vi "Set_tdms_properties.vi"(8 "Measurement Duration(s)":dbl=30.0 caption="Measurement Duration" format="%.3g", 11 "Temperature":string) -> (2 "Property Values":string[](array[string]), 3 "property names":string[](array[string])=["Temperature", "HV", "LV", "CH1 V/Div", "CH2 V/Div", "Trigger Level", "Trigger Source", "Coincidence"])   [LabVIEW 2019]
uses:
  SiPM_Tests_Global_Var.vi
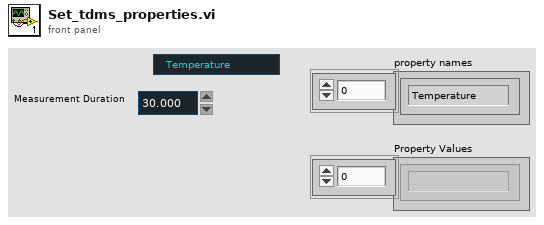
[diagram p1: front panel]
types:
  T1 = enum16{"Channel 1", "Channel 2", "Channel 3", "Channel 4", "D0", "D1", "D2", "D3", "D4", "D5", "D6", "D7", "D8", "D9", "D10", "D11", "D12", "D13", "D14", "D15", "External", "Power Line", "Waveform Generator"}
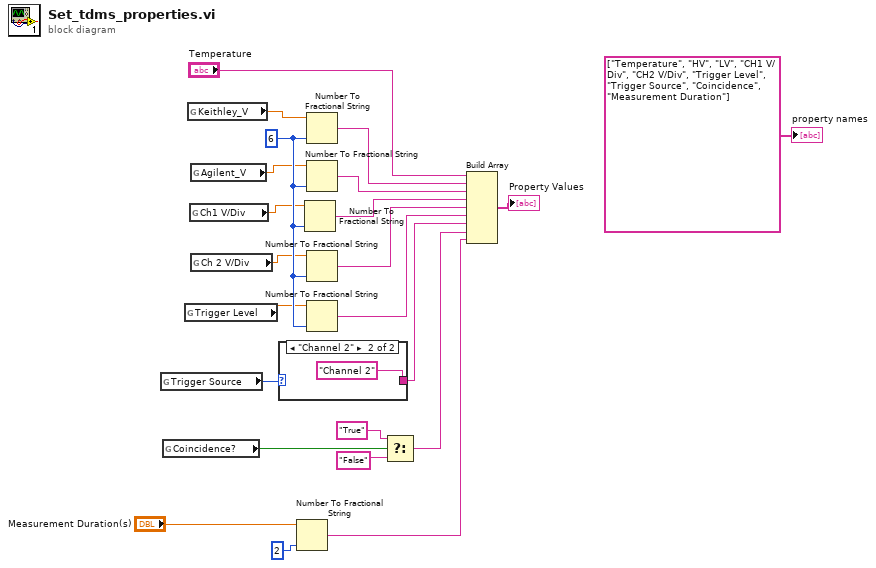
[diagram p0: block diagram]
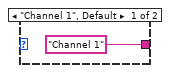
[diagram p2: hidden frame]
diagram:
  w14 = i16 6 ("precision (6)")
  n1 = global read "SiPM_Tests_Global_Var.vi" "Trigger Source"() -> (w16:T1)
  n2 = global read "SiPM_Tests_Global_Var.vi" "Coincidence?"() -> (w18:bool)
  n3 = global read "SiPM_Tests_Global_Var.vi" "Trigger Level"() -> (w13:dbl)
  n4 = global read "SiPM_Tests_Global_Var.vi" "Keithley_V"() -> (w4:dbl)
  n5 = global read "SiPM_Tests_Global_Var.vi" "Ch1 V/Div"() -> (w8:dbl)
  n6 = global read "SiPM_Tests_Global_Var.vi" "Agilent_V"() -> (w9:dbl)
  n7 = global read "SiPM_Tests_Global_Var.vi" "Ch 2 V/Div"() -> (w11:dbl)
  n8 = case shown="\"Channel 2\"" w16 {
    tunnel: ["Channel 1" "Channel 2"] -> w17
    frame "Channel 1", Default {
    }
    frame "Channel 2" {
    }
  }
  n9 = Number To Fractional String(number="Measurement Duration(s)", precision (6)=i16 2) -> (F-format string=w1:string)  [unwired: 2 in]
  n10 = Number To Fractional String(number=w8, precision (6)=w14) -> (F-format string=w10:string)  [unwired: 2 in]
  n11 = Number To Fractional String(number=w4, precision (6)=w14) -> (F-format string=w5:string)  [unwired: 2 in]
  n12 = Number To Fractional String(number=w9, precision (6)=w14) -> (F-format string=w6:string)  [unwired: 2 in]
  n13 = Number To Fractional String(number=w11, precision (6)=w14) -> (F-format string=w12:string)  [unwired: 2 in]
  n14 = Number To Fractional String(number=w13, precision (6)=w14) -> (F-format string=w15:string)  [unwired: 2 in]
  n15 = Select(t="True", s=w18, f="False") -> (s? t:f=w21:string)
  n16 = Build Array("Temperature", w5, w6, w10, w12, w15, w17, w21, w1) -> (→"Property Values":string[])
  "property names" <- string[] ["Temperature", "HV", "LV", "CH1 V/Div", "CH2 V/Div", "Trigger Level", "Trigger Source", "Coincidence", "Measurement Duration"] ("property names")
